vi "add_Image.vi"(4 "ROS Image":T1, 5 "msg in":string) -> (2 "msg out":string)   [LabVIEW 2010]
uses:
  <userlib>/ROSforLV_0.1/ROS/MessageBuilding/Primitives/subs/u32Scalar.vi
  <userlib>/ROSforLV_0.1/ROS/MessageBuilding/Primitives/subs/stringScalar.vi
  <userlib>/ROSforLV_0.1/ROS/MessageBuilding/Primitives/subs/u8Scalar.vi
  <userlib>/ROSforLV_0.1/ROS/MessageBuilding/Primitives/subs/u8Array.vi
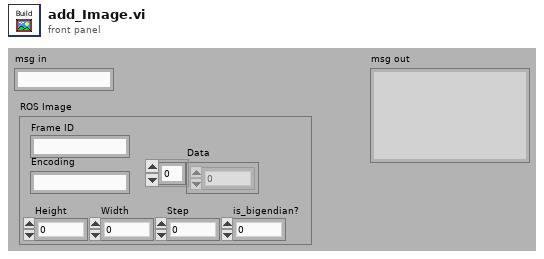
[diagram p1: front panel]
types:
  T1 = cluster{"Height":u32, "Width":u32, "is_bigendian?":u8, "Step":u32, "Data":u8[], "Encoding":string, "Frame ID":string}
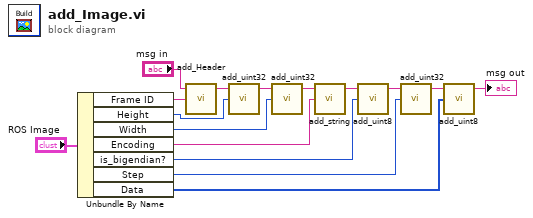
[diagram p0: block diagram]
diagram:
  n1 = Unbundle By Name("ROS Image") -> ("Frame ID"=w3:string, "Height"=w14:u32, "Width"=w12:u32, "Encoding"=w10:string, "is_bigendian?"=w8:u8, "Step"=w6:u32, "Data"=w4:u8[])
  n2 = call <userlib>:"add_Header.vi"("frame_id"=w3, "msg in"="msg in") -> ("msg out"=w15:string)  [unwired: 3 in]
  n3 = call-poly <userlib>:"add_uint32.vi"("Numeric"=w14, "msg in"=w15) -> ("msg out"=w13:string)  [unwired: 3 in]
  n4 = call-poly <userlib>:"add_uint32.vi"("Numeric"=w12, "msg in"=w13) -> ("msg out"=w11:string)  [unwired: 3 in]
  n5 = call-poly <userlib>:"add_string.vi"("String"=w10, "msg in"=w11) -> ("msg out"=w9:string)  [unwired: 3 in]
  n6 = call-poly <userlib>:"add_uint8.vi"("Numeric"=w8, "msg in"=w9) -> ("msg out"=w7:string)  [unwired: 3 in]
  n7 = call-poly <userlib>:"add_uint32.vi"("Numeric"=w6, "msg in"=w7) -> ("msg out"=w5:string)  [unwired: 3 in]
  n8 = call-poly <userlib>:"add_uint8.vi"("Array"=w4, "msg in"=w5) -> ("msg out"=→"msg out":string)  [unwired: 3 in]
